vi "Exit Program Event.vi"(8 "error in (no error)":errorcluster) -> (0 "error out":errorcluster)   [LabVIEW 2020, in "User Event.lvlib"]
doc: "For name actions"
uses:
  User Event.lvlib
  FGV Action.ctl
  Event Data.ctl
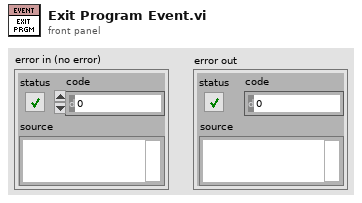
[diagram p1: front panel]
types:
  T1 = typedef "User Event.lvlib/Event Data.ctl" = enum16{"Exit Program"}
  T2 = typedef "User Event.lvlib/FGV Action.ctl" = enum16{"Create", "Get", "Destroy"}
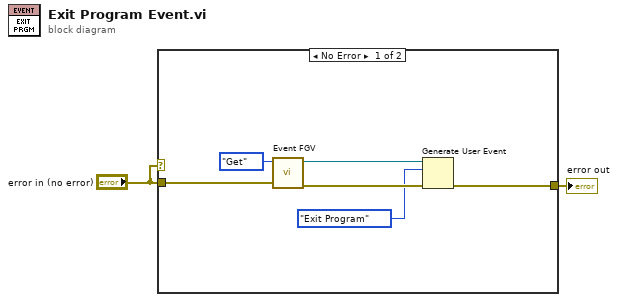
[diagram p0: block diagram]
diagram:
  n1 = case shown="No Error" "error in (no error)" {
    tunnel: "error in (no error)" -> [w7 w9]
    tunnel: [w3 w9] -> w1
    frame No Error {
      n2 = call "Event FGV.vi"("error in (no error)"=w7, "FGV Action"=FGV_Action."Get") -> ("error out"=w5:errorcluster, "Event Data"=w6:refnum<user-event>)  [unwired: 8 in]
      n3 = Generate User Event(user event=w6, event data cluster=Event_Data."Exit Program" ("event data"), error in=w5) -> (error out=w3:errorcluster)  [unwired: 1 in, 1 out]
    }
    frame Error {
    }
  }
  "error out" <- w1
